vi "Voice_coil_GB_var.vi"() -> ()   [LabVIEW 2020]
panel:
  in  "Voice coil string":string
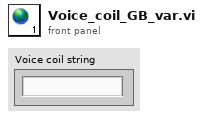
[diagram p1: front panel]
diagram:
